vi "Class instance - return.vi"() -> (0 "Class.lvclass":refnum<class "Class with PropertyNode.lvclass">)   [LabVIEW 2021, in "Class with PropertyNode.lvclass"]
uses:
  Class with PropertyNode.lvclass
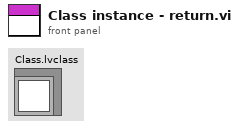
[diagram p1: front panel]
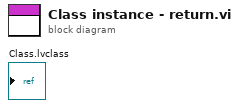
[diagram p0: block diagram]
diagram:
